vi "LR700 Parse Output.vi"(1 "String Read":string) -> (0 "?":dbl format="%.5e")   [LabVIEW 2019]
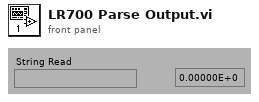
[diagram p1: front panel]
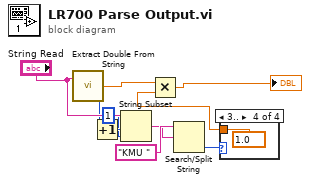
[diagram p0: block diagram]
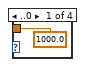
[diagram p2: hidden frame]
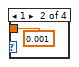
[diagram p3: hidden frame]
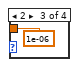
[diagram p4: hidden frame]
diagram:
  n1 = call "Extract Double From String.vi"("string"="String Read") -> ("floating pt. number"=w1:dbl, "end index"=w4:i32)  [unwired: 1 in, 1 out]
  n2 = Increment(x=w4) -> (x+1=w10:i32)
  n3 = String Subset(string="String Read", offset (0)=w10, length (rest)=1 ("length")) -> (substring=w6:string)
  n4 = Search/Split String(string="KMU ", search string/char (-)=w6) -> (offset of match=w8:i32)  [unwired: 1 in, 2 out]
  n5 = case shown="3.." w8 {
    tunnel: [1000.0 ("y") 0.001 ("y") 1e-06 ("y") 1.0 ("y")] -> w9
    frame ..0 {
    }
    frame 1 {
    }
    frame 2 {
    }
    frame 3.. {
    }
  }
  n6 = Multiply(x=w1, y=w9) -> (x*y=→"?":dbl)
